vi "parseFileString.vi"(8 "error in (no error)":errorcluster, 11 "IDLFile in":refnum<class "IDLFile.lvclass">) -> (0 "error out":errorcluster, 3 "IDLFile out":refnum<class "IDLFile.lvclass">)   [LabVIEW 2018, in "IDLFile.lvclass"]
uses:
  IDLFile.lvclass
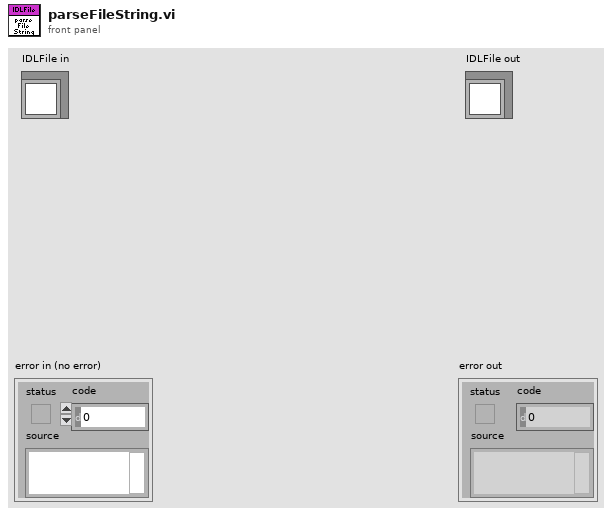
[diagram p1: front panel]
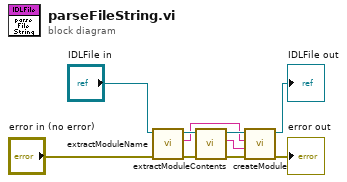
[diagram p0: block diagram]
diagram:
  n1 = call "extractModuleName.vi"("error in (no error)"="error in (no error)", "IDLFile in"="IDLFile in") -> ("error out"=w5:errorcluster, "moduleName"=w2:string, "IDLFile out"=w9:refnum<class "IDLFile.lvclass">)  [unwired: 7 in]
  n2 = call "extractModuleContents.vi"("error in (no error)"=w5, "IDLFile in"=w9) -> ("error out"=w4:errorcluster, "moduleContentsString"=w1:string, "IDLFile out"=w8:refnum<class "IDLFile.lvclass">)  [unwired: 7 in]
  n3 = call "createModule.vi"("error in (no error)"=w4, "moduleContentsString"=w1, "moduleName"=w2, "IDLFile in"=w8) -> ("error out"=→"error out":errorcluster, "IDLFile out"=→"IDLFile out":refnum<class "IDLFile.lvclass">)  [unwired: 6 in]
